vi "Get Default Log File Directory.vi"(8 "error in":errorcluster, 11 "Device Item Ref In":T1 format="%.0x") -> (0 "error out":errorcluster, 2 "Log File Directory String Array":string[](array[string]), 3 "Device Item Ref Out":T1 format="%.0x")   [LabVIEW 2019, in "Telemetry System Explorer.lvlib"]
uses:
  Telemetry System Explorer.lvlib
  <vilib>/NI VeriStand/Custom Device API/Custom Device Item Ref.ctl
  <vilib>/NI VeriStand/Custom Device API/Custom Device API.lvlib
  <vilib>/NI VeriStand/Custom Device Tools/Custom Device Utility Library/Custom Device Utility Library.lvlib
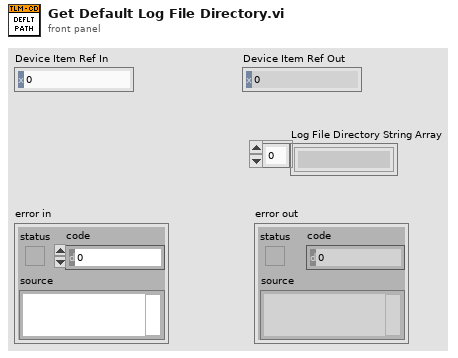
[diagram p1: front panel]
types:
  T1 = typedef "Custom Device API.lvlib/Custom Device Item Ref.ctl" = u64
  T2 = typedef "Custom Device API.lvlib/Custom Device Target Type.ctl" = enum16{"PharLap", "VxWorks", "Windows", "Linux_32_ARM", "Linux_x64"}
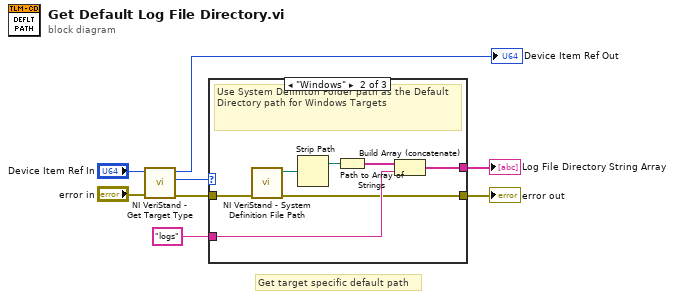
[diagram p0: block diagram]
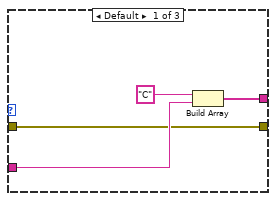
[diagram p2: hidden frame]
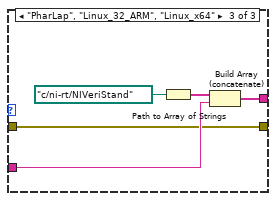
[diagram p3: hidden frame]
diagram:
  # "Get target specific default path"
  n1 = call <vilib>:"NI VeriStand - Get Target Type.vi"("error in (no error)"="error in", "Item Ref in"="Device Item Ref In") -> ("error out"=w3:errorcluster, "Target Type"=w6:T2, "Item Ref out"=→"Device Item Ref Out":T1)  [unwired: 7 in]
  n2 = case shown="\"Windows\"" w6 {
    tunnel: [w11 w18 w23] -> w8
    tunnel: "logs" -> [w12 w19 w24]
    tunnel: w3 -> [w10 w17 w21]
    tunnel: [w10 w16 w21] -> w2
    frame Default {
      n3 = Build Array("C" ("element"), w12) -> (w11:string[])
    }
    frame "Windows" {
      # "Use System Definiton Folder path as the Default Directory path for Windows Targets"
      n4 = call <vilib>:"NI VeriStand - System Definition File Path.vi"("error in (no error)"=w17) -> ("error out"=w16:errorcluster, "SDF path"=w15:path)  [unwired: 9 in]
      n5 = Strip Path(path=w15) -> (stripped path=w14:path)  [unwired: 1 out]
      n6 = Path to Array of Strings(0:w14) -> (2:w13:string[])  [unwired: 1 out]
      n7 = Build Array (concatenate)(w13, w19) -> (w18:string[])
    }
    frame "PharLap", "Linux_32_ARM", "Linux_x64" {
      n8 = Path to Array of Strings(0:path "c:/ni-rt/NIVeriStand" ("path")) -> (2:w20:string[])  [unwired: 1 out]
      n9 = Build Array (concatenate)(w20, w24) -> (w23:string[])
    }
  }
  "Log File Directory String Array" <- w8
  "error out" <- w2
